vi "RevertToSelf.vi"(8 "error in (no error)":errorcluster, 11 "Impersonate in":refnum<class "LogonUser.lvclass">) -> (0 "error out":errorcluster, 3 "Impersonate out":refnum<class "LogonUser.lvclass">)   [LabVIEW 2018, in "LogonUser.lvclass"]
doc: "©2019\nWiebe Walstra\nwww.carya.nl"
uses:
  LogonUser.lvclass
  advapi32.dll
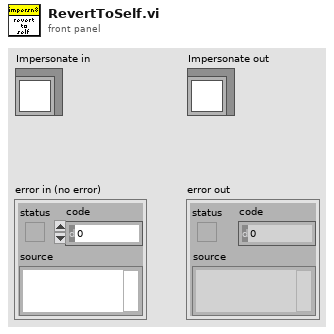
[diagram p1: front panel]
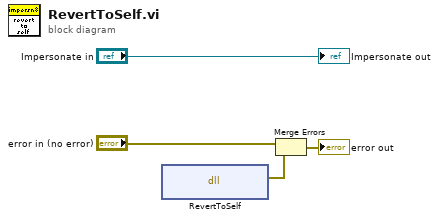
[diagram p0: block diagram]
diagram:
  n1 = dll-call lib="advapi32.dll" fn="RevertToSelf"() -> (error out=w1:errorcluster)  [unwired: 4 in, 1 out]
  n2 = Merge Errors("error in (no error)", w1) -> (→"error out":errorcluster)
  "Impersonate out" <- "Impersonate in"
